vi "remove_string_elements.vi"(10 "Array in":string[](array[string]), 11 "spreadsheet string":string) -> (3 "Array out":string[](array[string]))   [LabVIEW 2015]
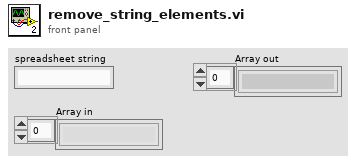
[diagram p1: front panel]
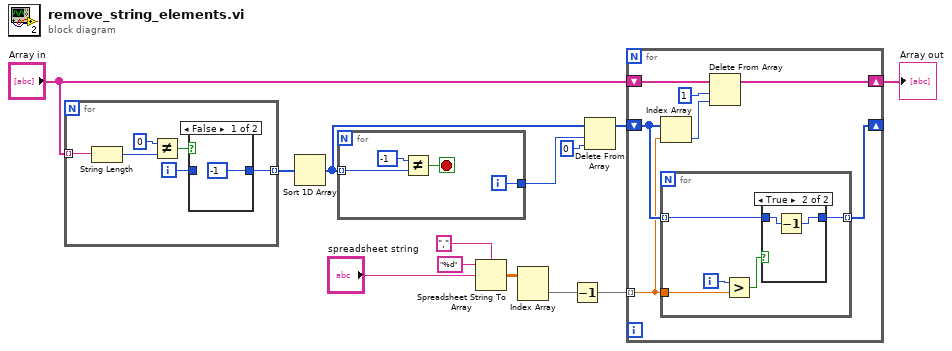
[diagram p0: block diagram]
diagram:
  n1 = for {
    tunnel: "Array in" -> [w17] mode=indexing
    tunnel: [w14] -> w1 mode=indexing
    i -> [w15]
    n2 = String Length(string=w17) -> (length=w19:i32)
    n3 = Not Equal?(x=0, y=w19) -> (x != y?=w16:bool)
    n4 = case shown="False" w16 {
      tunnel: w15 -> [_ w21]
      tunnel: [-1 w21] -> w14
      frame False {
      }
      frame True {
      }
    }
  }
  n5 = Sort 1D Array(array=w1) -> (sorted array=w3:i32[])
  n6 = for {
    tunnel: w3 -> [w23] mode=indexing
    tunnel: [w22] -> w2
    i -> [w22]
    stop <- w24 stop-if-true
    n7 = Not Equal?(x=-1, y=w23) -> (x != y?=w24:bool)
  }
  n8 = Spreadsheet String To Array(delimiter (Tab)=",", format string="%d", spreadsheet string="spreadsheet string") -> (array=w8:dbl[][])  [unwired: 1 in]
  n9 = Index Array(array=w8) -> (element=w10:dbl[])  [unwired: 2 in]
  n10 = Decrement(x=w10) -> (x-1=w11:dbl[])
  n11 = Delete From Array(array=w3, length=w2, index=0) -> (array with subset deleted=w9:i32[])  [unwired: 1 out]
  n12 = for {
    tunnel: w11 -> [w27] mode=indexing
    shift-right: [w26] -> _
    shift-left: w9 -> [w28]
    shift-right: [w29] -> w12
    shift-left: "Array in" -> [w30]
    n13 = Index Array(array=w28, index=w27) -> (element=w31:i32)
    n14 = for {
      tunnel: w28 -> [w37] mode=indexing
      tunnel: w27 -> [w36]
      tunnel: [w33] -> w26 mode=indexing
      i -> [w35]
      n15 = Greater?(x=w35, y=w36) -> (0:w34:bool)
      n16 = case shown="True" w34 {
        tunnel: w37 -> [w38 w40]
        tunnel: [w38 w39] -> w33
        frame False {
        }
        frame True {
          n17 = Decrement(x=w40) -> (x-1=w39:i32)
        }
      }
    }
    n18 = Delete From Array(array=w30, length=1, index=w31) -> (array with subset deleted=w29:string[])  [unwired: 1 out]
  }
  "Array out" <- w12
